vi "Setup TS.vi"(8 "error in":errorcluster, 11 "Test Stand in":refnum<class "Cryo Sep Test Stand.lvclass">) -> (0 "error out":errorcluster, 3 "Test Stand out":refnum<class "Cryo Sep Test Stand.lvclass">)   [LabVIEW 2019, in "Test Stands.lvlib" / "Cryo Sep Test Stand.lvclass"]
uses:
  Cryo Sep Test Stand.lvclass
  C:/Users/krio/Documents/LV_Projects/test-stand/App/Generic Test Stand/Generic Test Stand.lvclass
  DAC/DeepU/TC Temperature/DAC TC Temp DeepU.lvclass
  C:/Users/krio/Documents/LV_Projects/test-stand/App/DAC/DAC.lvclass
  DAC/DAC.lvclass/DAC.ctl
  Generic Test Stand/Generic Test Stand.lvclass/Generic Test Stand.ctl
  Generic Test Stand/Generic Test Stand.lvclass
  DAC/DAC.lvclass
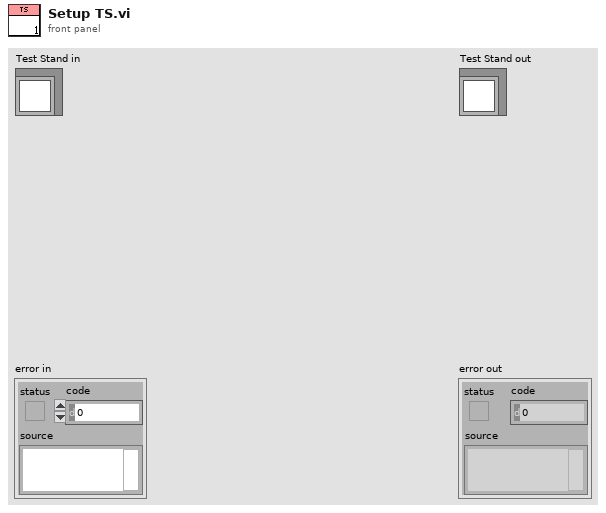
[diagram p1: front panel]
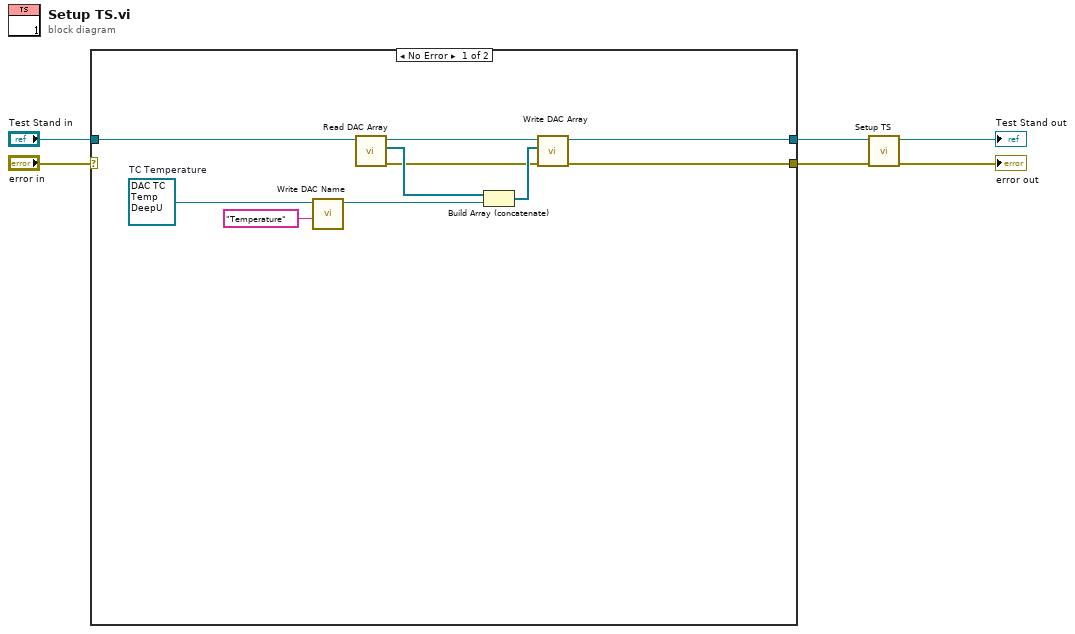
[diagram p0: block diagram]
diagram:
  n1 = case shown="No Error" "error in" {
    selector: "error in" -> [_ w17]
    tunnel: "Test Stand in" -> [w16 w18]
    tunnel: [w10 w18] -> w2
    tunnel: [w9 w17] -> w1
    frame No Error {
      w7 = refnum<class "DAC TC Temp DeepU.lvclass"> refnum  # TC Temperature
      n2 = call "Write DAC Name.vi"("DAC Name"="Temperature", "DAC in"=w7) -> ("DAC out"=w8:refnum<class "DAC TC Temp DeepU.lvclass">)  [unwired: 8 in, 1 out]
      n3 = call "Read DAC Array.vi"("Generic Test Stand in"=w16) -> ("error out"=w12:errorcluster, "DAC Array"=w15:refnum<class "DAC.lvclass">[], "Generic Test Stand out"=w14:refnum<class "Cryo Sep Test Stand.lvclass">)  [unwired: 8 in]
      n4 = Build Array (concatenate)(w15, w8) -> (w13:refnum<class "DAC.lvclass">[])
      n5 = call "Write DAC Array.vi"("error in (no error)"=w12, "DAC Array"=w13, "Generic Test Stand in"=w14) -> ("error out"=w9:errorcluster, "Generic Test Stand out"=w10:refnum<class "Cryo Sep Test Stand.lvclass">)  [unwired: 7 in]
    }
    frame Error {
    }
  }
  n6 = call-parent "Setup TS.vi"("error in (no error)"=w1, "Generic Test Stand in"=w2) -> ("error out"=→"error out":errorcluster, "Generic Test Stand out"=→"Test Stand out":refnum<class "Cryo Sep Test Stand.lvclass">)  [unwired: 8 in]
